vi "StopCapture.vi"(0 "object in":refnum<class "Hamamatsu.lvclass">, 5 "error in (no error)":errorcluster) -> (14 "object out":refnum<class "Hamamatsu.lvclass">, 19 "error out":errorcluster)   [LabVIEW 2021, in "Hamamatsu.lvclass"]
uses:
  Hamamatsu.lvclass
  Hamamatsu.lvclass/Hamamatsu.ctl
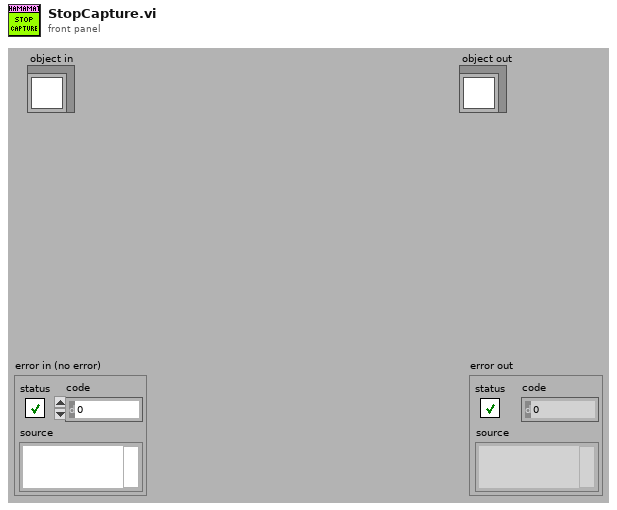
[diagram p1: front panel]
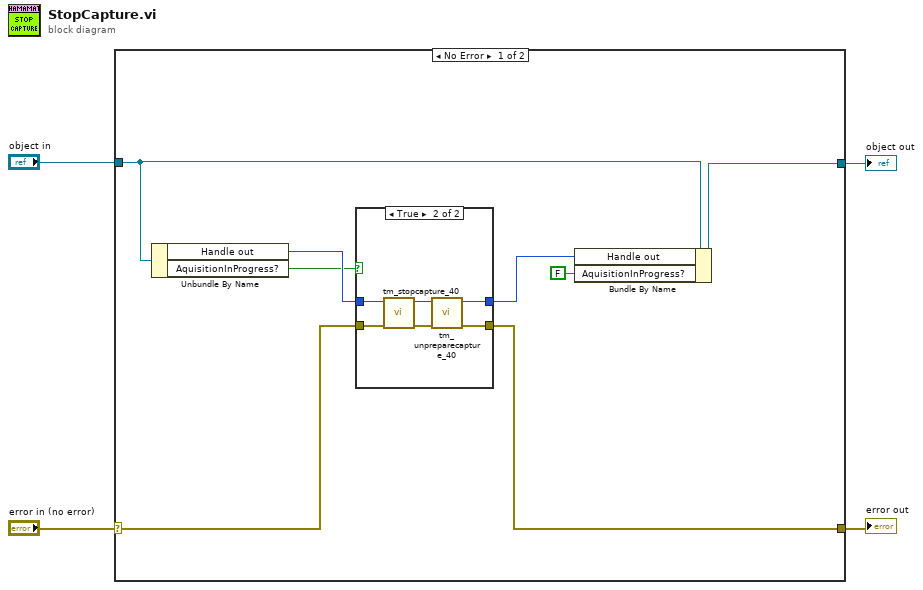
[diagram p0: block diagram]
diagram:
  n1 = case shown="No Error" "error in (no error)" {
    selector: "error in (no error)" -> [w9 w22]
    tunnel: [w8 w22] -> w3
    tunnel: [w11 w21] -> w1
    tunnel: "object in" -> [w12 w21]
    frame No Error {
      n2 = Unbundle By Name(w12) -> ("Handle out"=w10:u32, "AquisitionInProgress?"=w5:bool)
      n3 = case shown="True" w5 {
        tunnel: w10 -> [w14 w18]
        tunnel: w9 -> [w13 w17]
        tunnel: [w13 w16] -> w8
        tunnel: [w14 w15] -> w7
        frame False {
        }
        frame True {
          n4 = call <userlib>:"tm_stopcapture_40.vi"("error in (no error)"=w17, "Handle in"=w18) -> ("error out"=w19:errorcluster, "Handle out"=w20:u32)  [unwired: 8 in]
          n5 = call <userlib>:"tm_unpreparecapture_40.vi"("error in (no error)"=w19, "Handle in"=w20) -> ("error out"=w16:errorcluster, "Handle out"=w15:u32)  [unwired: 8 in]
        }
      }
      n6 = Bundle By Name(cluster=w12, "Handle out"=w7, "AquisitionInProgress?"=FALSE) -> (w11:refnum<class "Hamamatsu.lvclass">)
    }
    frame Error {
    }
  }
  "error out" <- w3
  "object out" <- w1
